vi "Update Selected.vi"(8 "error in (no error)":errorcluster, 10 "Array":bool[](array[boolean]), 11 "Test Selector in":refnum<class "Test Selector.lvclass">) -> (0 "error out":errorcluster, 3 "Test Selector out":refnum<class "Test Selector.lvclass">)   [LabVIEW 2019, in "Test Selector.lvlib" / "Test Selector.lvclass"]
uses:
  Test Selector.lvclass
  Test Selector.lvclass/Test Selector.ctl
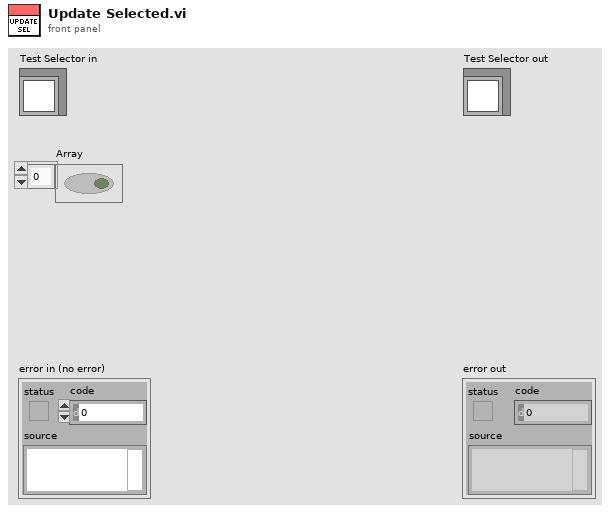
[diagram p1: front panel]
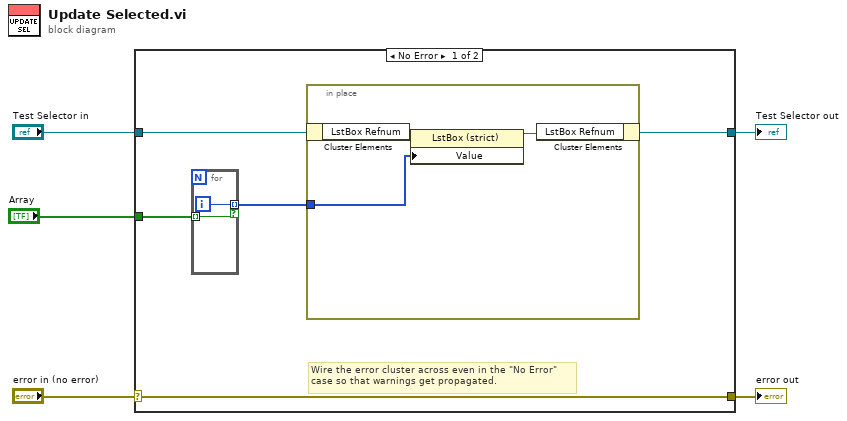
[diagram p0: block diagram]
diagram:
  n1 = case shown="No Error" "error in (no error)" {
    selector: "error in (no error)" -> [w10 w17]
    tunnel: [w10 w17] -> w4
    tunnel: [w7 w16] -> w2
    tunnel: "Test Selector in" -> [w8 w16]
    tunnel: "Array" -> [w9 _]
    frame No Error {
      # "Wire the error cluster across even in the \"No Error\"\ncase so that warnings get propagated."
      n2 = for {
        tunnel: w9 -> [w14] mode=indexing
        tunnel: [w15] -> w6 mode=indexing if=w14
        i -> [w15]
      }
      n3 = in-place {
        in-place-border: w6 -> [w11]
        n4 = in-place-cluster #1(w8) -> ("LstBox Refnum"=w13:refnum<vi>)
        n5 = property class="LstBox (strict)"(reference=w13, "Value"=w11) -> (reference out=w12:refnum<vi>)  [unwired: 1 in, 1 out]
        n6 = in-place-cluster #1("LstBox Refnum"=w12) -> (w7:refnum<class "Test Selector.lvclass">)
      }
    }
    frame Error {
    }
  }
  "error out" <- w4
  "Test Selector out" <- w2
